vi "Initialise.vi"(8 "Size":u16 format="%04x", 9 "Offset":u16 format="%04x", 10 "Data":u8[](array[numeric]), 11 "Table":refnum<vi>) -> (3 "Hex Viewer":refnum<class "Hex Viewer.lvclass">)   [LabVIEW 2021, in "Hex Viewer.lvclass"]
uses:
  Hex Viewer.lvclass
  <vilib>/Utility/miscctls.llb/LVRowAndColumnTypeDef.ctl
  <vilib>/Utility/miscctls.llb/LVRowAndColumnUnsignedTypeDef.ctl
  Hex Viewer.lvclass/Hex Viewer.ctl
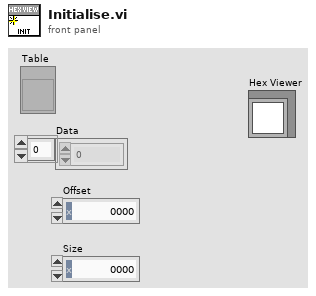
[diagram p1: front panel]
types:
  T1 = typedef "LVRowAndColumnUnsignedTypeDef.ctl" = cluster{"Row":u32, "Column":u32}
  T2 = typedef "LVRowAndColumnTypeDef.ctl" = cluster{"Row":i32, "Column":i32}
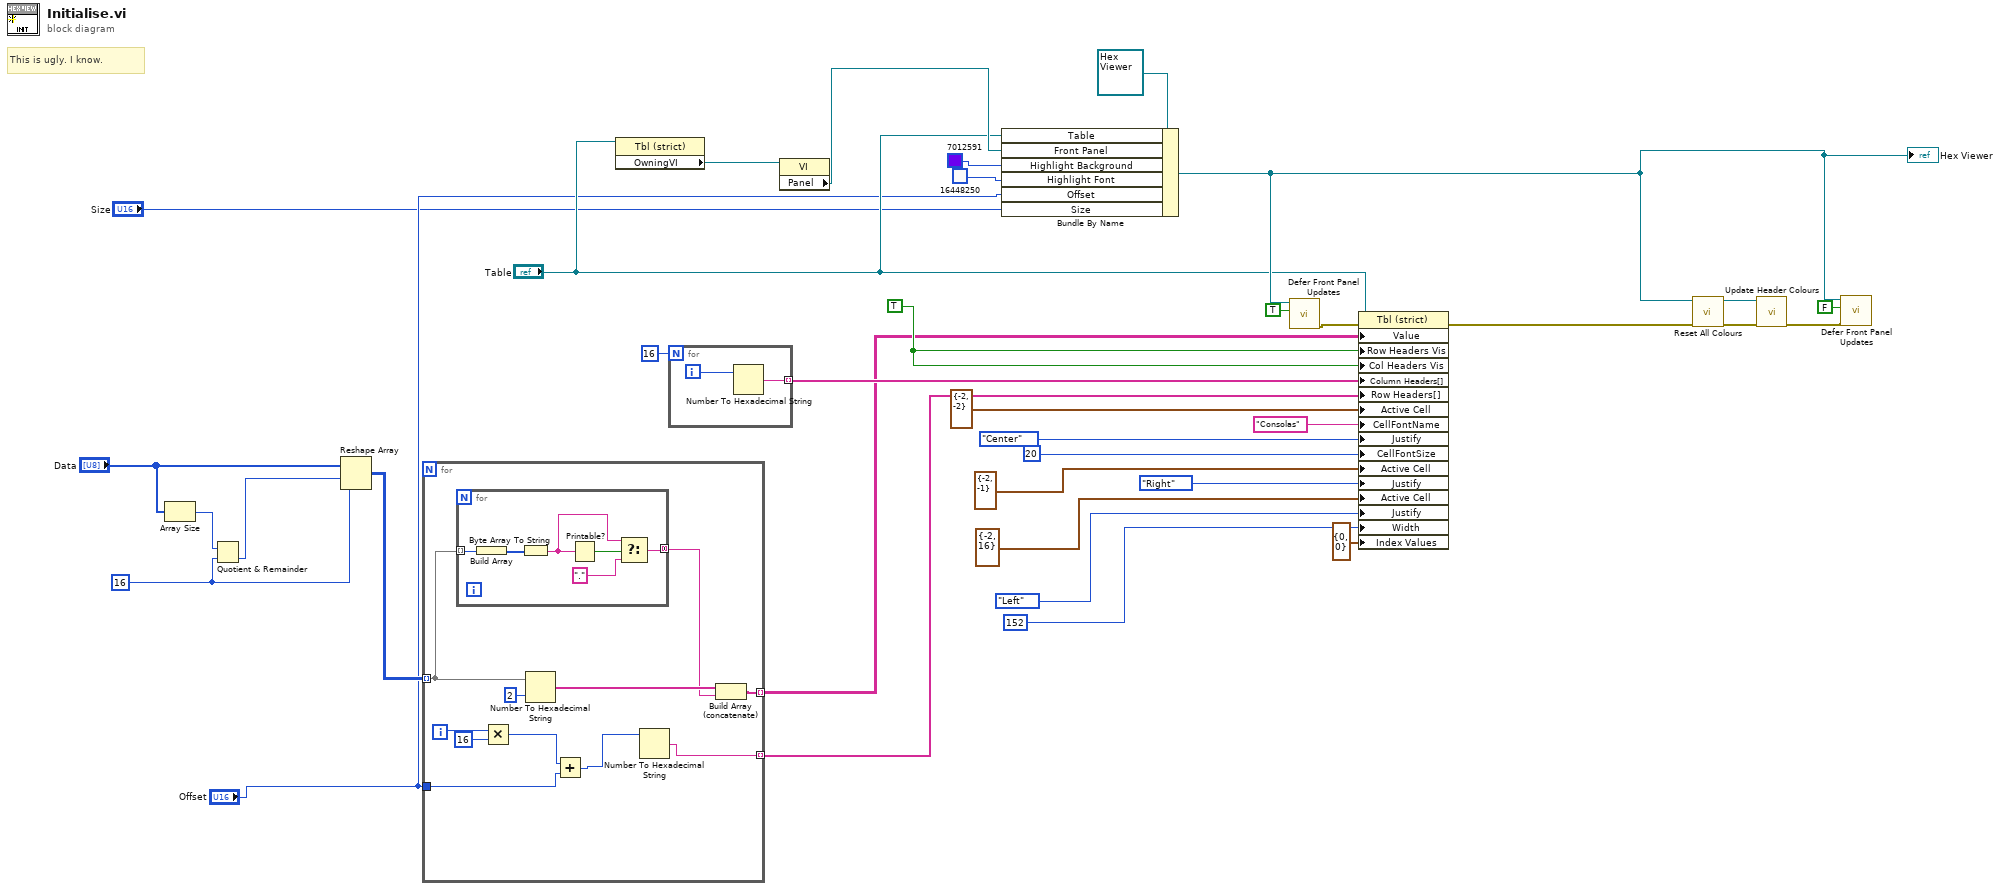
[diagram p0: block diagram]
diagram:
  w35 = TRUE ("Visible Items:Row Headers Visible")
  w19 = 16
  # "This is ugly. I know."
  n1 = Array Size(array="Data") -> (size(s)=w20:i32)
  n2 = Quotient & Remainder(x=w20, y=w19) -> (floor(x/y)=w18:i32)  [unwired: 1 out]
  n3 = Reshape Array("Data", w18, w19) -> (w31:u8[][])
  n4 = for {
    tunnel: w31 -> [w40] mode=indexing
    tunnel: [w44] -> w32 mode=indexing
    tunnel: [w41] -> w14 mode=indexing
    tunnel: "Offset" -> [w38]
    i -> [w46]
    n5 = for {
      tunnel: w40 -> [w52] mode=indexing
      tunnel: [w47] -> w39 mode=concatenating
      n6 = Build Array(w52) -> (w51:u8[])
      n7 = Byte Array To String(unsigned byte array=w51) -> (string=w49:string)
      n8 = Printable?(1:w49) -> (0:w50:bool)
      n9 = Select(t=w49, s=w50, f=".") -> (s? t:f=w47:string)
    }
    n10 = Multiply(x=w46, y=16) -> (x*y=w37:i32)
    n11 = Number To Hexadecimal String(1:i16 2 ("width (-)"), 2:w40) -> (0:w42:string[])
    n12 = Add(x=w37, y=w38) -> (x+y=w36:i32)
    n13 = Number To Hexadecimal String(2:w36) -> (0:w44:string)  [unwired: 1 in]
    n14 = Build Array (concatenate)(w42, w39) -> (w41:string[])
  }
  n15 = property class="Tbl (strict)"(reference="Table") -> ("OwningVI"=w12:refnum<vi>)  [unwired: 1 in, 2 out]
  n16 = for {
    N: 16 -> [_]
    tunnel: [w53] -> w33 mode=indexing
    i -> [w54]
    n17 = Number To Hexadecimal String(2:w54) -> (0:w53:string)  [unwired: 1 in]
  }
  n18 = property class="VI"(reference=w12) -> ("Panel"=w11:refnum<vi>)  [unwired: 1 in, 2 out]
  n19 = Bundle By Name(cluster=refnum<class "Hex Viewer.lvclass"> refnum ("Hex Viewer.lvclass"), "Table"="Table", "Front Panel"=w11, "Highlight Background"=u32 7012591 ("Color Box"), "Highlight Font"=u32 16448250 ("Color Box 2"), "Offset"="Offset", "Size"="Size") -> (w6:refnum<class "Hex Viewer.lvclass">)
  "Hex Viewer" <- w6
  n20 = call "Defer Front Panel Updates.vi"("Defer"=TRUE, "Hex Viewer in"=w6) -> ("error out"=w10:errorcluster)  [unwired: 9 in]
  n21 = property class="Tbl (strict)"(reference="Table", error in=w10, "Value"=w14, "Row Headers Vis"=w35, "Col Headers Vis"=w35, "Column Headers[]"=w33, "Row Headers[]"=w32, "Active Cell"=T2 {"Row"=-2, "Column"=-2} ("Active Cell:Active Cell"), "CellFontName"="Consolas" ("Active Cell:Cell Font:Name"), "Justify"=enum16{"Left", "Center", "Right"}."Center" ("Active Cell:Cell Justification"), "CellFontSize"=u32 20 ("Active Cell:Cell Font:Size"), "Active Cell"=T2 {"Row"=-2, "Column"=-1} ("Active Cell:Active Cell"), "Justify"=enum16{"Left", "Center", "Right"}."Right" ("Active Cell:Cell Justification"), "Active Cell"=T2 {"Row"=-2, "Column"=16} ("Active Cell:Active Cell"), "Justify"=enum16{"Left", "Center", "Right"}."Left" ("Active Cell:Cell Justification"), "Width"=u32 152 ("Active Cell:Cell Size:Width"), "Index Values"=T1 {"Row"=0, "Column"=0}) -> (error out=w9:errorcluster)  [unwired: 1 out]
  n22 = call "Reset All Colours.vi"("error in (no error)"=w9, "Hex Viewer in"=w6) -> ("error out"=w13:errorcluster)  [unwired: 9 in]
  n23 = call "Update Header Colours.vi"("error in (no error)"=w13, "Hex Viewer in"=w6) -> ("error out"=w7:errorcluster)  [unwired: 9 in]
  n24 = call "Defer Front Panel Updates.vi"("error in (no error)"=w7, "Defer"=FALSE, "Hex Viewer in"=w6) -> ()  [unwired: 8 in, 1 out]
